vi "Cancel_Query.vi"(8 "error in (no error)":errorcluster, 11 "Postgres Connector In":refnum<class "Postgres Connector.lvclass">) -> (0 "error out":errorcluster)   [LabVIEW 2019, in "PG_LIB.lvlib" / "Postgres Connector.lvclass"]
doc: "This VI is used to cancel a query. It open a TCP connection and cancel the actual query. There is no need to close the connection after because the server will close it automatically.\ns"
uses:
  Postgres Connector.lvclass
  Postgres Connector.lvclass/Postgres Connector.ctl
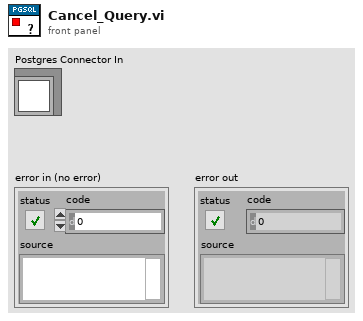
[diagram p1: front panel]
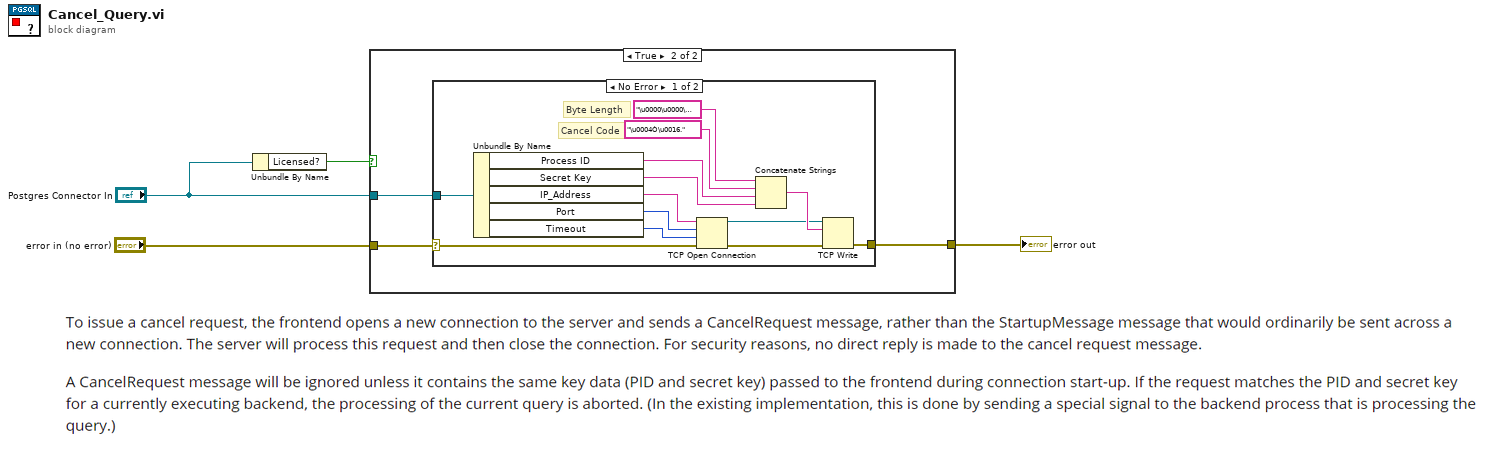
[diagram p0: block diagram]
diagram:
  n1 = Unbundle By Name("Postgres Connector In") -> ("Licensed?"=w1:bool)
  n2 = case shown="True" w1 {
    tunnel: "Postgres Connector In" -> [_ w8]
    tunnel: [w5 w7] -> w4
    tunnel: "error in (no error)" -> [w5 w6]
    frame False {
    }
    frame True {
      n3 = case shown="No Error" w6 {
        selector: w6 -> [w11 w22]
        tunnel: w8 -> [w14 _]
        tunnel: [w12 w22] -> w7
        frame No Error {
          # "Cancel Code"
          # "Byte Length"
          n4 = Unbundle By Name(w14) -> ("Process ID"=w10:string, "Secret Key"=w9:string, "IP_Address"=w21:string, "Port"=w20:u16, "Timeout"=w19:i32)
          n5 = TCP Open Connection(address=w21, remote port or service name=w20, timeout ms (60000)=w19, error in (no error)=w11) -> (connection ID=w13:refnum<k5>, error out=w18:errorcluster)  [unwired: 1 in]
          n6 = Concatenate Strings("\u0000\u0000\u0000\u0010", "\u0004Ò\u0016." ("string"), w10, w9) -> (w15:string)
          n7 = TCP Write(connection ID=w13, data in=w15, error in (no error)=w18) -> (error out=w12:errorcluster)  [unwired: 1 in, 2 out]
        }
        frame Error {
        }
      }
    }
  }
  "error out" <- w4
